vi "Spawned Program.vi"() -> ()   [LabVIEW 2018]
panel:
  in  "stop":bool
  out "String":string
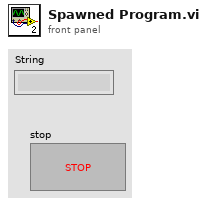
[diagram p1: front panel]
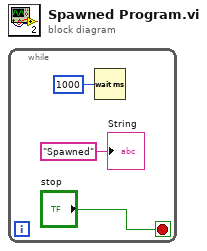
[diagram p0: block diagram]
diagram:
  n1 = while {
    stop <- "stop" stop-if-true
    n2 = Wait (ms)(milliseconds to wait=u32 1000) -> ()  [unwired: 1 out]
    "String" <- "Spawned" ("String")
  }
